vi "WriteToFile.vi"(8 "error in":errorcluster, 9 "Log Prefix":string="VNALog", 10 "VNACluster In":T3={"Value"=0.0, "GUI Data Cluster"={"S11"=FALSE, "S21"=FALSE, "S12"=FALSE, "S22"=FALSE, "S11Meas"=enum."Log-magnitude (dB)", "S21Meas"=enum."Log-magnitude (dB)", "S12Meas"=enum."Log-magnitude (dB)", "S22Meas"=enum."Log-magnitude (dB)"}, "Timing"={"Last Operation"=0.0, "Stop @ T/B"=FALSE, "Last Temp"=0.0, "Last Mag"=0.0, "Ramp Param"={"End T (K)"=0.0, "Delta T (K)"=0.0, "End B (T)"=0.0, "Delta B (T)"=0.0}, "LastOp?"=FALSE, "FirstOp?"=FALSE}, "Measurements"=[], "Hardware"={"VNA TCP Con"=refnum, "VNA TCP Port"=5025, "Global T VAR"="", "Global B VAR"=""}, "Operation"={"Operation Mode"=enum."Logging", "Log Folder"=path "", "Measure Mode"=enum."Deltat"}}, 11 "TerminalIn":T1) -> (0 "error out":errorcluster, 2 "VNACluster Out":T3={"Value"=0.0, "GUI Data Cluster"={"S11"=FALSE, "S21"=FALSE, "S12"=FALSE, "S22"=FALSE, "S11Meas"=enum."Log-magnitude (dB)", "S21Meas"=enum."Log-magnitude (dB)", "S12Meas"=enum."Log-magnitude (dB)", "S22Meas"=enum."Log-magnitude (dB)"}, "Timing"={"Last Operation"=0.0, "Stop @ T/B"=FALSE, "Last Temp"=0.0, "Last Mag"=0.0, "Ramp Param"={"End T (K)"=0.0, "Delta T (K)"=0.0, "End B (T)"=0.0, "Delta B (T)"=0.0}, "LastOp?"=FALSE, "FirstOp?"=FALSE}, "Measurements"=[], "Hardware"={"VNA TCP Con"=refnum, "VNA TCP Port"=5025, "Global T VAR"="", "Global B VAR"=""}, "Operation"={"Operation Mode"=enum."Logging", "Log Folder"=path "", "Measure Mode"=enum."Deltat"}}, 3 "TerminalOut":T1)   [LabVIEW 2021]
uses:
  Data_Cluster.ctl
  Measurement_Cluster.ctl
  Mode_Enum.ctl
  Library/TerminalDef.ctl
  <vilib>/Utility/config.llb/Config Data RefNum.ctl
  <vilib>/Utility/file.llb/Write Delimited Spreadsheet (DBL).vi
  Library/LibDan.lvlib
  <vilib>/Utility/config.llb/NI_LVConfig.lvlib
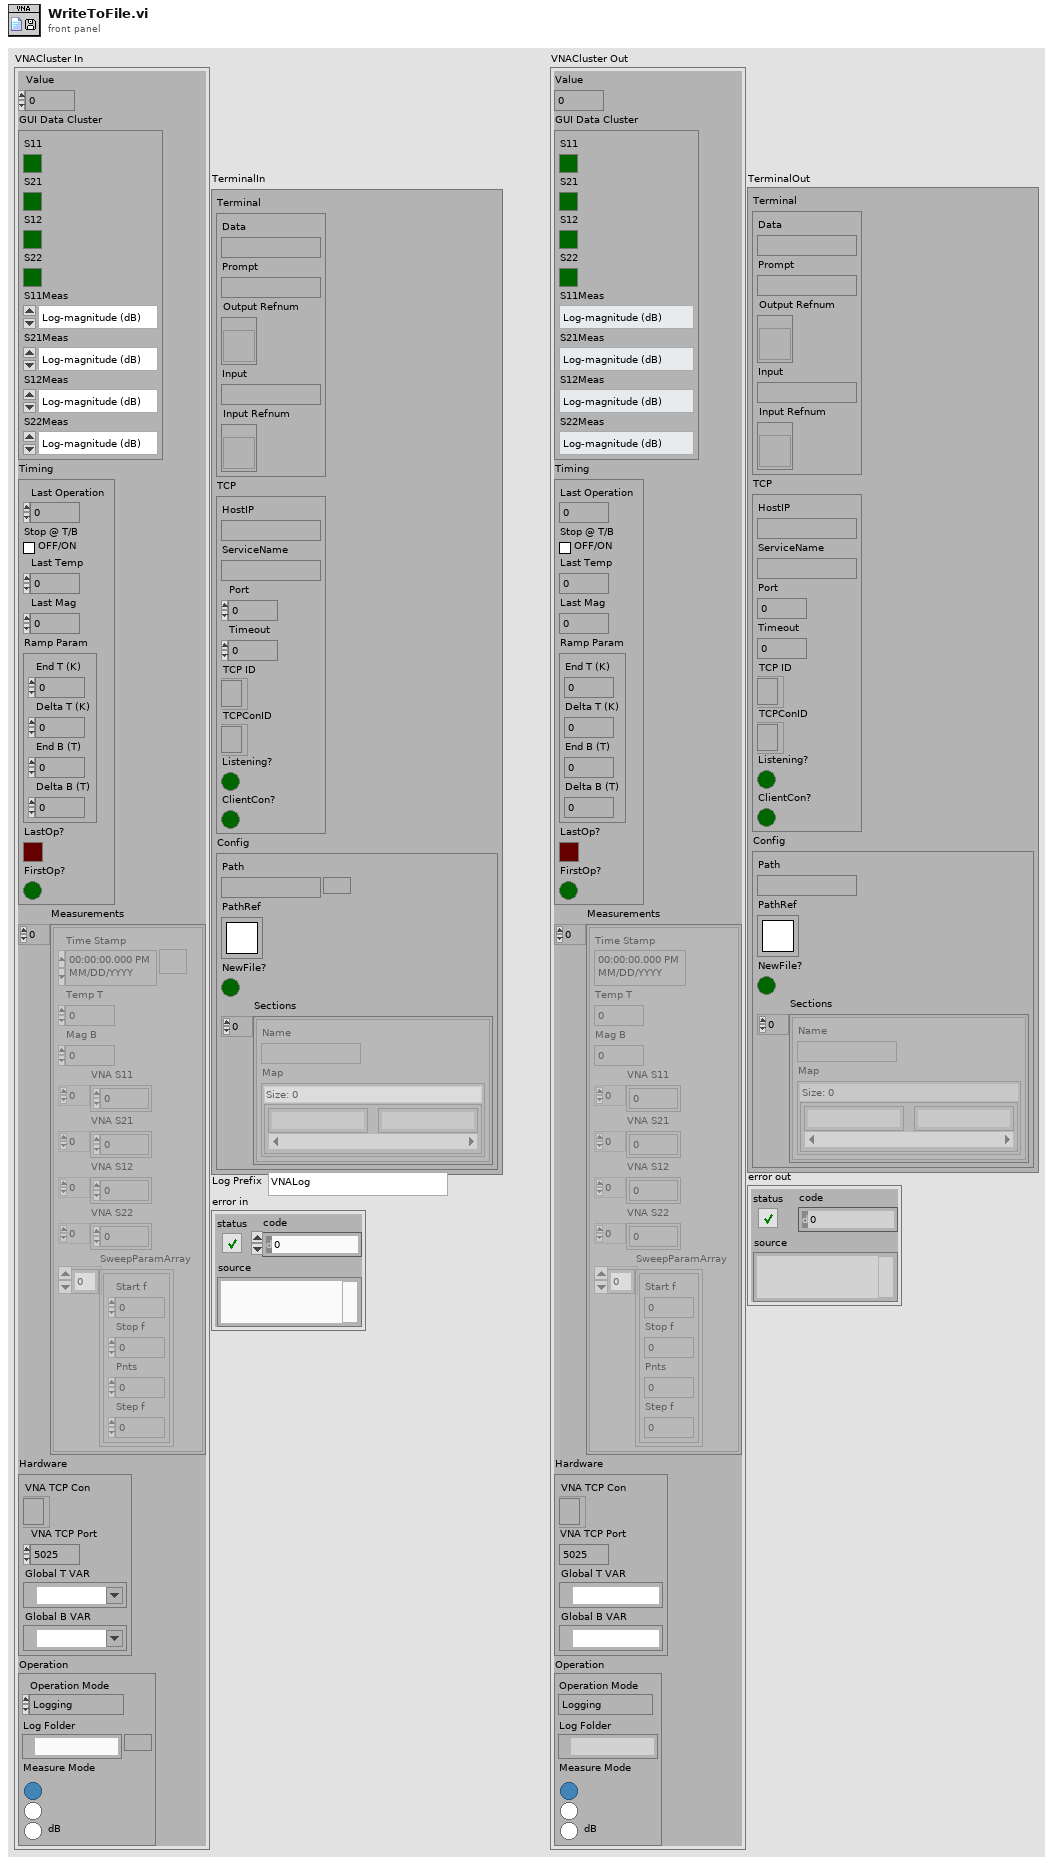
[diagram p1: front panel]
types:
  T1 = typedef "LibDan.lvlib/TerminalDef.ctl" = cluster{"Terminal":cluster{"Data":string, "Prompt":string, "Output Refnum":refnum<vi>, "Input":string, "Input Refnum":refnum<vi>}, "TCP":cluster{"HostIP":string, "ServiceName":string, "Port":u16, "Timeout":i32, "TCP ID":refnum<k5>, "TCPConID":refnum<k5>, "Listening?":bool, "ClientCon?":bool}, "Config":cluster{"Path":path, "PathRef":T2, "NewFile?":bool, "Sections":cluster{"Name":string, "Map":map{string, string}}[]}}
  T2 = typedef "NI_LVConfig.lvlib/Config Data RefNum.ctl" = refnum<k1>
  T3 = typedef "Data_Cluster.ctl" = cluster{"Value":dbl, "GUI Data Cluster":cluster{"S11":bool, "S21":bool, "S12":bool, "S22":bool, "S11Meas":enum16{"Log-magnitude (dB)", "Linear magnitude", "Phase (deg)", "Time Domain", "Real", "Imaginary", "Group Delay", "Polarlinear"}, "S21Meas":enum16{"Log-magnitude (dB)", "Linear magnitude", "Phase (deg)", "Time Domain", "Real", "Imaginary", "Group Delay", "Polarlinear"}, "S12Meas":enum16{"Log-magnitude (dB)", "Linear magnitude", "Phase (deg)", "Time Domain", "Real", "Imaginary", "Group Delay", "Polarlinear"}, "S22Meas":enum16{"Log-magnitude (dB)", "Linear magnitude", "Phase (deg)", "Time Domain", "Real", "Imaginary", "Group Delay", "Polarlinear"}}, "Timing":cluster{"Last Operation":dbl, "Stop @ T/B":bool, "Last Temp":dbl, "Last Mag":dbl, "Ramp Param":cluster{"End T (K)":dbl, "Delta T (K)":dbl, "End B (T)":dbl, "Delta B (T)":dbl}, "LastOp?":bool, "FirstOp?":bool}, "Measurements":T4[], "Hardware":cluster{"VNA TCP Con":refnum<k5>, "VNA TCP Port":i32, "Global T VAR":refnum<k21>, "Global B VAR":refnum<k21>}, "Operation":cluster{"Operation Mode":T5, "Log Folder":path, "Measure Mode":enum32{"Deltat", "DeltaT", "dB"}}}
  T4 = typedef "Measurement_Cluster.ctl" = cluster{"Time Stamp":timestamp, "Temp T":dbl, "Mag B":dbl, "VNA S11":dbl[], "VNA S21":dbl[], "VNA S12":dbl[], "VNA S22":dbl[], "SweepParamArray":cluster{"Start f":dbl, "Stop f":dbl, "Pnts":i32, "Step f":dbl}[]}
  T5 = typedef "Mode_Enum.ctl" = enum16{"Logging", "Idle-Off", "Idle"}
  T6 = cluster{"Start f":dbl, "Stop f":dbl, "Pnts":i32, "Step f":dbl}[]
  T7 = cluster{"Start f":dbl, "Stop f":dbl, "Pnts":i32, "Step f":dbl}
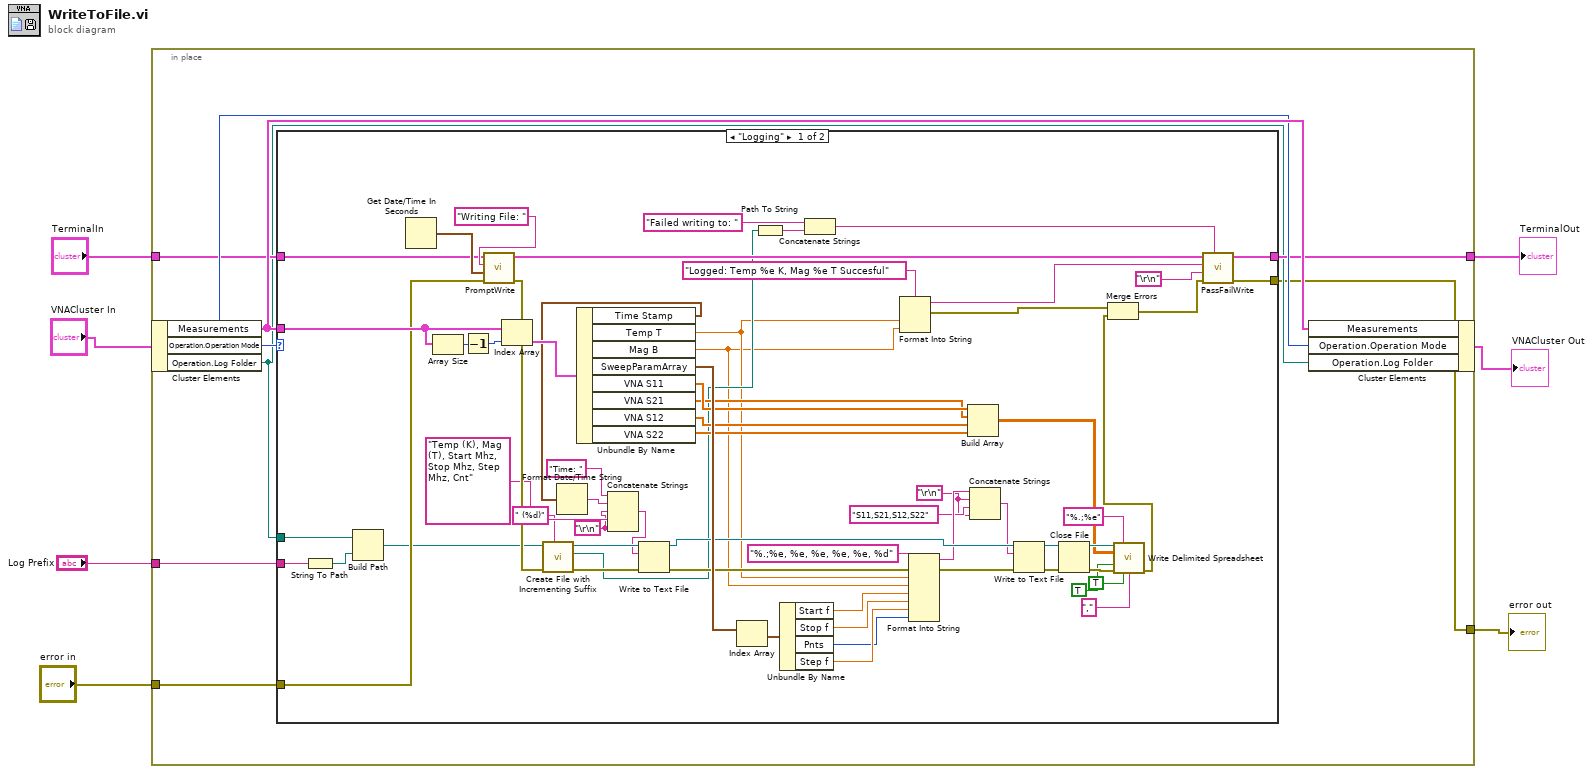
[diagram p0: block diagram]
diagram:
  n1 = in-place {
    in-place-border: "TerminalIn" -> [w13]
    in-place-border: [w12] -> w4
    in-place-border: "Log Prefix" -> [w10]
    in-place-border: "error in" -> [w9]
    in-place-border: [w8] -> w1
    n2 = in-place-cluster #1("VNACluster In") -> ("Measurements"=w15:T4[], "Operation.Operation Mode"=w14:T5, "Operation.Log Folder"=w11:path)
    n3 = case shown="\"Logging\"" w14 {
      tunnel: w15 -> [w77 _]
      tunnel: w13 -> [w72 w81]
      tunnel: [w71 w81] -> w12
      tunnel: w11 -> [w70 _]
      tunnel: w10 -> [w68 _]
      tunnel: w9 -> [w66 w80]
      tunnel: [w39 w80] -> w8
      frame "Logging" {
        w31 = "\r\n"
        w51 = "\r\n"
        n4 = String To Path(string=w68) -> (path=w69:path)
        n5 = Build Path(base path=w70, name or relative path=w69) -> (appended path=w29:path)
        n6 = Get Date/Time In Seconds() -> (seconds since 1Jan1904=w74:timestamp)
        n7 = Array Size(array=w77) -> (size(s)=w79:i32)
        n8 = Decrement(x=w79) -> (x-1=w78:i32)
        n9 = call "PromptWrite.vi"("error in"=w66, "time"=w74, "string"="Writing File: ", "TerminalIn"=w72) -> ("error out"=w67:errorcluster, "TerminalOut"=w27:T1)  [unwired: 6 in]
        n10 = Index Array(array=w77, index=w78) -> (element=w76:T4)
        n11 = call <vilib>:"Create File with Incrementing Suffix.vi"("format string (\" (%d)\")"=" (%d)" ("format string (\" (%d)\")"), "error in (no error)"=w67, "file path"=w29) -> ("error out"=w62:errorcluster, "actual path"=w24:path, "refnum out"=w65:refnum<file>)  [unwired: 6 in]
        n12 = Unbundle By Name(w76) -> ("Time Stamp"=w34:timestamp, "Temp T"=w21:dbl, "Mag B"=w20:dbl, "SweepParamArray"=w64:T6, "VNA S11"=w45:dbl[], "VNA S21"=w44:dbl[], "VNA S12"=w43:dbl[], "VNA S22"=w42:dbl[])
        n13 = Format Date/Time String(seconds (now)=w34) -> (date/time string=w32:string)  [unwired: 2 in]
        n14 = Concatenate Strings("Time: ", w32, w31, "Temp (K), Mag (T), Start Mhz, Stop Mhz, Step Mhz, Cnt" ("initial string"), w31) -> (w36:string)
        n15 = Write to Text File(file (use dialog)=w65, text=w36, error in=w62) -> (refnum out=w54:refnum<file>, error out=w60:errorcluster)  [unwired: 1 in, 1 out]
        n16 = Index Array(array=w64) -> (element=w63:T7)  [unwired: 1 in]
        n17 = Path To String(path=w24) -> (string=w25:string)
        n18 = Unbundle By Name(w63) -> ("Start f"=w59:dbl, "Stop f"=w58:dbl, "Pnts"=w56:i32, "Step f"=w57:dbl)
        n19 = Concatenate Strings("Failed writing to: " ("FailString"), w25) -> (w23:string)
        n20 = Format Into String(format string="Logged: Temp %e K, Mag %e T Succesful", w21, w20) -> (resulting string=w19:string, error out=w17:errorcluster)  [unwired: 2 in]
        n21 = Format Into String(format string="%.;%e, %e, %e, %e, %e, %d", error in=w60, w21, w20, w59, w58, w57, w56) -> (resulting string=w53:string, error out=w55:errorcluster)  [unwired: 1 in]
        n22 = Build Array(w45, w44, w43, w42) -> (w41:dbl[][])
        n23 = Concatenate Strings(w53, w51, "S11,S21,S12,S22" ("text"), w51) -> (w50:string)
        n24 = Write to Text File(file (use dialog)=w54, text=w50, error in=w55) -> (refnum out=w49:refnum<file>, error out=w48:errorcluster)  [unwired: 1 in, 1 out]
        n25 = Close File(refnum=w49, error in=w48) -> (path=w47:path, error out=w46:errorcluster)
        n26 = call-poly <vilib>:"Write Delimited Spreadsheet.vi"("file path (dialog if empty)"=w47, "format (%.3f)"="%.;%e", "2D data"=w41, "append to file? (new file:F)"=TRUE, "error in (no error)"=w46, "transpose? (no:F)"=TRUE, "delimiter (\\t)"="," ("delimiter (\\t)")) -> ("error out"=w18:errorcluster)  [unwired: 7 in, 1 out]
        n27 = Merge Errors(w17, w18) -> (w16:errorcluster)
        n28 = call "PassFailWrite.vi"("FailString"=w23, "error in"=w16, "End"="\r\n", "PassString"=w19, "TerminalIn"=w27) -> ("error out"=w39:errorcluster, "TerminalOut"=w71:T1)  [unwired: 5 in]
      }
      frame "Idle-Off", Default {
      }
    }
    n29 = in-place-cluster #1("Measurements"=w15, "Operation.Operation Mode"=w14, "Operation.Log Folder"=w11) -> (→"VNACluster Out":T3)
  }
  "TerminalOut" <- w4
  "error out" <- w1
